vi "Subvi AO Pockels.vi"(2 "AO":refnum<k21>="Connector1/AO0", 7 "Ext trigger":bool, 8 "Scaling Factor":refnum<k21>="SCALING1", 9 "FIFO In":refnum<k21>="GALVO1") -> ()   [LabVIEW 2017]
uses:
  <vilib>/Platform/TimedLoop/XDataNode/timing_clust.ctl
  <vilib>/Platform/TimedLoop/XDataNode/nitl_modes.ctl
  <vilib>/Platform/TimedLoop/XDataNode/wakeup.ctl
  <vilib>/rvi/Emulation/niFpgaSctlEmulationGetInTimedLoop.vi
  <vilib>/rvi/Emulation/niFpgaEmulationReportErrorSimple.vi
  <vilib>/rvi/Emulation/niFpgaGetClockAttributes.vi
  <vilib>/rvi/Emulation/niFpgaCriticalErrorInLSC.vi
  Detector/GV frameclock.vi
  Detector/GV frame counter.vi
  <vilib>/rvi/DataTransferAndStorage/Container/Common/niFpgaContainerExecOnDevCompGetState.vi
  <vilib>/rvi/Emulation/niFpgaEmulationIsFPGAContextNoSignature.vi
  <vilib>/rvi/DataTransferAndStorage/Container/Common/niFpgaContainerGetUniqueNameForEmu.vi
  <vilib>/rvi/Emulation/niFpgaProcessEmulError.vi
  <vilib>/rvi/errors/nirviReportUnexpectedCaseInternalError (U32).vi
  <vilib>/rvi/Memory/Memory_Emulation/niFpgaMemoryEmulationCacheClearOnFirstRun.vi
  <vilib>/rvi/Memory/Memory_Emulation/nirvimemoryEmulationManagerCache_MakeExclusive.vi
  <vilib>/rvi/Memory/Memory_Emulation/niFpgaMemoryEmulationValidateCache.vi
  <vilib>/rvi/Memory/Memory_Emulation/nirvimemoryEmulationManagerCache_InsertValue.vi
  <vilib>/Utility/error.llb/Clear Errors.vi
  <vilib>/rvi/Memory/Memory_Emulation/nirvimemoryEmulationManagerCache_ReleaseExclusive.vi
  <vilib>/rvi/Memory/Memory_Emulation/nirvimemoryEmulationManagerCache_GetValue.vi
  <vilib>/rvi/Memory/Memory_Emulation/nirvimemoryEmulationManagerCache_SetValue.vi
  <vilib>/rvi/Emulation/niFpgaSctlEmulationResourceMgr.vi
  <vilib>/rvi/eio/common/nirviEmuTemplateMethod_errors.vi
  <vilib>/Platform/TimedLoop/XDataNode/XDataNode.xnode
  <vilib>/rvi/DataTransferAndStorage/Container/XNode/niFpgaContainer.xnode
  <vilib>/rvi/Memory/Memory_Emulation/niFpgaMemoryEmulationRefIn.vi
  <vilib>/eio/EIONode/EIONode.xnode
  <vilib>/Platform/TimedLoop/XDataNode/XDNodeRunTimeDep.lvlib
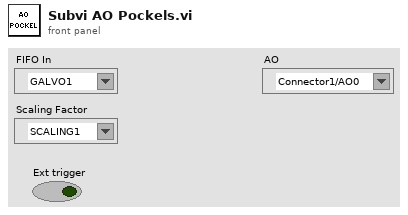
[diagram p1: front panel]
types:
  T1 = typedef "XDNodeRunTimeDep.lvlib/timing_clust.ctl" = cluster{"Expected End [f-1]":u64, "Actual End [f-1]":u64, "Finished Late? [f-1]":bool, "Expected End [i-1]":u64, "Actual End [i-1]":u64, "Finished Late? [i-1]":bool, "Expected Start [i]":u64, "Actual Start [i]":u64, "Expected Start [f]":u64, "Actual Start [f]":u64, "Source Name":string, "Structure Name":string, "Period":i64, "Deadline":i64, "Offset":i64, "Start":i64, "Priority":i32, "Timeout":i32, "Mode":T2, "Wakeup Reason":T3, "Error":errorcluster, "Source Type":string, "Secondary Source Type":string, "Global End Time":u64, "Global Start Time":u64, "Frame Duration":u64, "Iteration Duration":u64, "Assigned CPU":i32, "I/O Scan Engine Mode":u32}
  T2 = typedef "XDNodeRunTimeDep.lvlib/nitl_modes.ctl" = enum32{"No Change", "Process missed periods, maintain original phase", "Discard missed periods, maintain original phase", "Process missed periods, ignore original phase", "Discard missed periods, ignore original phase"}
  T3 = typedef "XDNodeRunTimeDep.lvlib/wakeup.ctl" = enum32{"Normal", "Aborted", "Asynchronous wakeup", "Timing source error", "Timed loop error", "Timeout"}
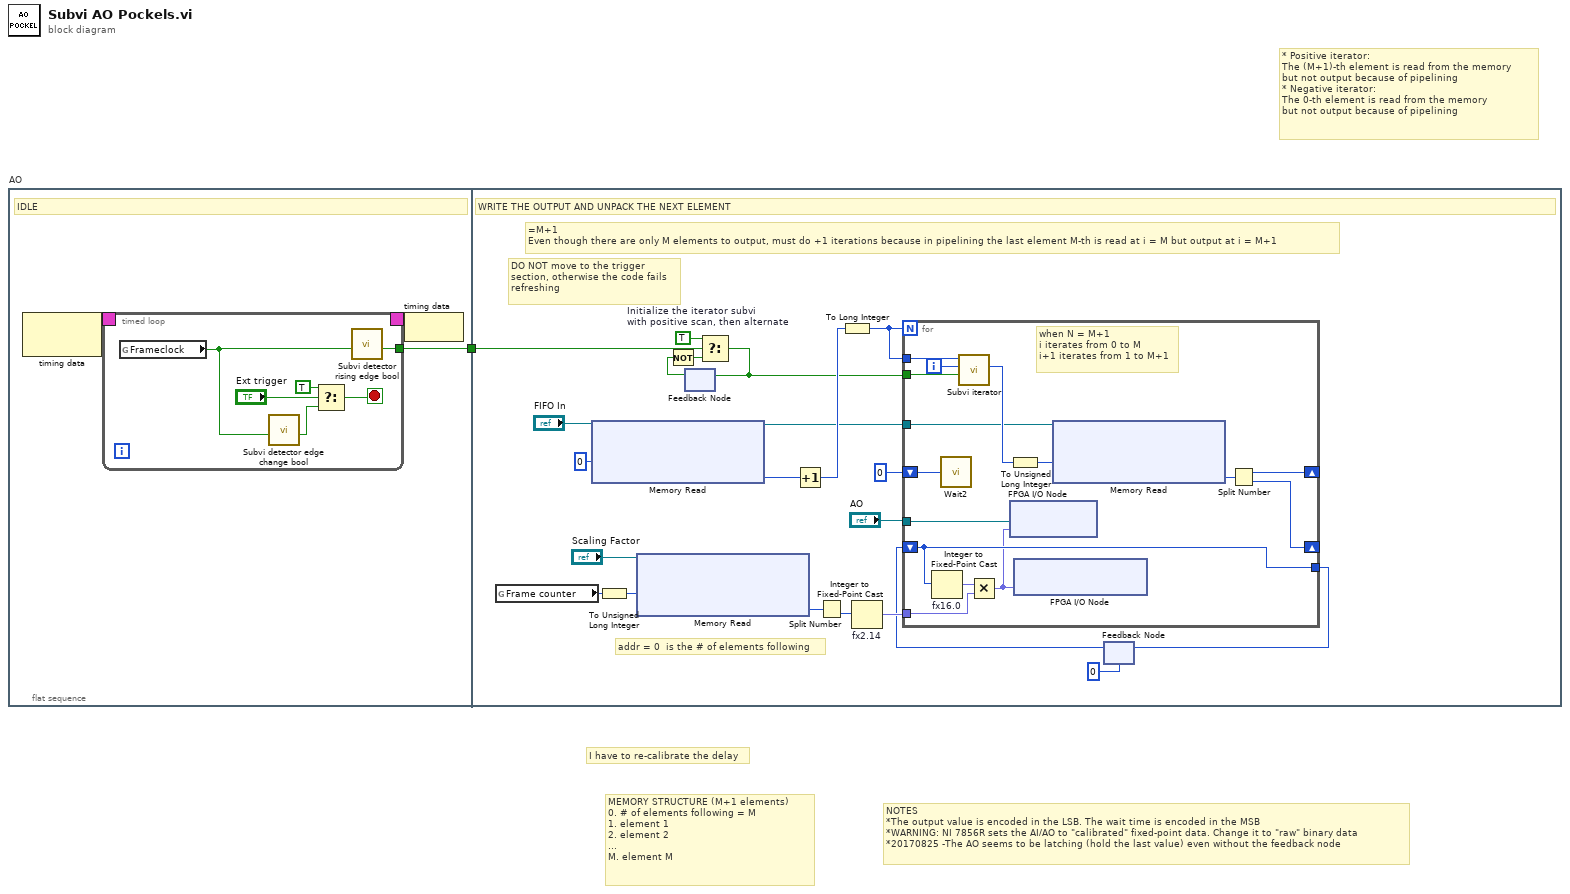
[diagram p0: block diagram]
diagram:
  # "* Positive iterator:\nThe (M+1)-th element is read from the memory \nbut not output because of pipelining\n* Negative iterator:\nThe 0-th element is read from the memory \nbut not output because of pipelining"
  # "MEMORY STRUCTURE (M+1 elements)\n0. # of elements following = M\n1. element 1\n2. element 2\n...\nM. element M"
  # "I have to re-calibrate the delay"
  # "NOTES\n*The output value is encoded in the LSB. The wait time is encoded in the MSB\n*WARNING: NI 7856R sets the AI/AO to \"calibrated\" fixed-point data. Change it to \"raw\" binary data\n*20170825 -The AO seems to be latching (hold the last value) even without the feedback node"
  n1 = flat-sequence "AO" {
    tunnel: [w2] -> w1
    tunnel: w1 -> [w23]
    frame #0 {
      # "IDLE"
      n2 = node-c288() -> (w4:T1)  [unwired: 1 in]
      n3 = timed-loop {
        timing: w4 -> [_]
        timing-out: [_] -> w3
        tunnel: [w6] -> w2
        stop <- w9 stop-if-true
        n4 = global read "GV frameclock.vi" "Frameclock"() -> (w5:bool)
        n5 = call "Subvi detector edge change bool.vi"("Input"=w5) -> ("Output"=w8:bool)  [unwired: 8 in]
        n6 = Select(t=TRUE, s="Ext trigger", f=w8) -> (s? t:f=w9:bool)
        n7 = call "Subvi detector rising edge bool.vi"("Input"=w5) -> ("Output"=w6:bool)  [unwired: 10 in]
      }
      n8 = node-c288(w3) -> ()
    }
    frame #1 {
      # "addr = 0  is the # of elements following"
      # "DO NOT move to the trigger\nsection, otherwise the code fails\nrefreshing"
      # "=M+1\nEven though there are only M elements to output, must do +1 iterations because in pipelining the last element M-th is read at i = M but output at i = M+1"
      # "WRITE THE OUTPUT AND UNPACK THE NEXT ELEMENT"
      n9 = global read "GV frame counter.vi" "Frame counter"() -> (w17:u8)
      n10 = xnode ("Memory Read")("Address"=u32 0, "Memory In"="FIFO In") -> ("Data"=w31:u32, "Memory Out"=w30:refnum<k21>)
      n11 = To Unsigned Long Integer(number=w17) -> (unsigned 32bit integer=w16:u32)
      n12 = xnode ("Memory Read")("Address"=w16, "Memory In"="Scaling Factor") -> ("Data"=w18:u32)  [unwired: 1 out]
      n13 = feedback #1() -> (w27:bool)  [unwired: 1 in]
      n14 = Not(x=w27) -> (.not. x?=w26:bool)
      n15 = Select "Initialize the iterator subvi\nwith positive scan, then alternate"(t=TRUE, s=w23, f=w26) -> (s? t:f=w24:bool)
      n16 = feedback-in #1(w24) -> ()
      n17 = Increment(x=w31) -> (x+1=w34:u32)
      n18 = Split Number(x=w18) -> (lo(x)=w22:u16)  [unwired: 1 out]
      n19 = To Long Integer(number=w34) -> (32bit integer=w33:i32)
      n20 = Integer to Fixed-Point Cast "fx2.14"(integer=w22) -> (fixed-point=w21:fxp<+,16,2>)  [unwired: 1 in]
      n21 = feedback #2(u16 0) -> (w20:u16)
      n22 = for {
        N: w33 -> [_]
        shift-right: [w49] -> _
        shift-left: u16 0 -> [w48]
        shift-right: [w38] -> _
        shift-left: w20 -> [w41]
        tunnel: [w41] -> w35
        tunnel: w33 -> [w45]
        tunnel: w30 -> [w44]
        tunnel: w24 -> [w43]
        tunnel: w21 -> [w42]
        tunnel: "AO" -> [w37]
        i -> [w46]
        # "when N = M+1\ni iterates from 0 to M\ni+1 iterates from 1 to M+1"
        n23 = Integer to Fixed-Point Cast "fx16.0"(integer=w41) -> (fixed-point=w40:fxp<+/-,16,16>)  [unwired: 1 in]
        n24 = call "Wait2"("Count(Ticks)"=w48) -> ()  [unwired: 1 out]
        n25 = call "Subvi iterator.vi"("Set increase"=w43, "Iterator in"=w46, "Nmax"=w45) -> ("Iterator out"=w47:i32)  [unwired: 7 in, 1 out]
        n26 = Multiply(x=w40, y=w42) -> (x*y=w39:fxp<+/-,32,18>)
        n27 = To Unsigned Long Integer(number=w47) -> (unsigned 32bit integer=w51:u32)
        n28 = xnode ("FPGA I/O Node")("I/O Item"=w39, "FPGA I/O In"=w37) -> ()  [unwired: 1 out]
        n29 = xnode "FPGA I/O Node"("Connector1/AO7"=w39) -> ()  [unwired: 1 in, 1 out]
        n30 = xnode ("Memory Read")("Address"=w51, "Memory In"=w44) -> ("Data"=w50:u32)  [unwired: 1 out]
        n31 = Split Number(x=w50) -> (hi(x)=w49:u16, lo(x)=w38:u16)
      }
      n32 = feedback-in #2(w35) -> ()
    }
  }
